vi "Store Configuration Parameters.vi"(8 "error in (no error)":errorcluster, 10 "refnum":T1, 11 "Example Configuration Dialog in":refnum<class "Motor Configuration.lvclass">) -> (0 "error out":errorcluster, 2 "refnum out":T1, 3 "Example Configuration Dialog out":refnum<class "Motor Configuration.lvclass">)   [LabVIEW 2016, in "Hardware.lvlib" / "Motor.lvlib" / "Motor Configuration.lvclass"]
uses:
  <userlib>/Common Components/Hardware/Motor/Motor Config/Motor Configuration.lvclass
  <vilib>/Utility/config.llb/Config Data RefNum.ctl
  <userlib>/Common Components/Hardware/Motor/Motor/Motor.lvclass/Motor.ctl
  <userlib>/Common Components/Hardware/Abstract Hardware/Hardware.lvclass/Hardware.ctl
  <userlib>/Common Components/Hardware/DevInfo/DevInfo.lvclass/DevInfo.ctl
  <userlib>/Common Components/Hardware/Abstract Hardware/Read Label.vi
  <userlib>/Common Components/Hardware/Abstract Hardware/Read DevInfo.vi
  <userlib>/Common Components/Hardware/DevInfo/Read HW Type.vi
  <userlib>/Common Components/Hardware/DevInfo/Read Device Name.vi
  <userlib>/Common Components/Hardware/DevInfo/Read COMM Address.vi
  <userlib>/Common Components/Hardware/DevInfo/Read Sub-COMM Address.vi
  <userlib>/Common Components/Hardware/Motor/Motor/Motor.lvclass
  C:/Program Files (x86)/National Instruments/LabVIEW 2016/user.lib/Common Components/Hardware/Abstract Hardware/Hardware.lvclass
  <userlib>/Common Components/Hardware/Motor/Motor Config/Accessors/Read Motor Obj.vi
  <userlib>/Common Components/Hardware/DevInfo/DevInfo.lvclass
  <vilib>/Utility/config.llb/NI_LVConfig.lvlib
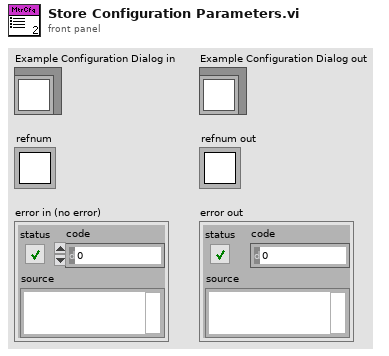
[diagram p1: front panel]
types:
  T1 = typedef "NI_LVConfig.lvlib/Config Data RefNum.ctl" = refnum<k1>
  T2 = typedef "Hardware.lvlib/Motor.lvlib/Motor.lvclass/Motor_Parameters.ctl" = cluster{"closed loop?":bool, "encoder?":bool, "min speed":dbl, "max speed":dbl, "acc time (s)":dbl, "dec time (s)":dbl, "unit mode":enum16{"motor pulses", "real world"}, "motor pulses per revolution":dbl, "display units per motor rev":dbl, "encoder units ratio":dbl, "display unit":string, "display precision":u8, "soft limit min":dbl, "soft limit max":dbl, "Max No. of pull-ins":u8, "Limit+":bool, "Limit+ Logic":enum16{"Low", "High"}, "Limit+ Mode":enum16{"Stop immediately", "Decelerate to Stop"}, "Limit-":bool, "Limit- Logic":enum16{"Low", "High"}, "Limit- Mode":enum16{"Stop immediately", "Decelerate to Stop"}, "Limit+ Sensor ID":enum16{"N/A", "S1", "S2", "S3"}, "Limit- Sensor ID":enum16{"N/A", "S1", "S2", "S3"}, "backlash Compensation":dbl, "soft offset":dbl, "backlash option":enum16{"None", "arriving in + direction", "arriving in - direction"}, "encoder type":enum16{"Linear", "Rotary"}}
  T3 = typedef "Hardware.lvlib/Motor.lvlib/Motor.lvclass/Home Params.ctl" = cluster{"Home Mode":T4, "Home Dir":T5, "Home Pos Shift":dbl}
  T4 = typedef "Hardware.lvlib/Motor.lvlib/Motor.lvclass/Home Mode.ctl" = enum16{"EZ+EL", "EZ only"}
  T5 = typedef "Hardware.lvlib/Motor.lvlib/Motor.lvclass/Home Dir.ctl" = enum16{"negative-", "positive+"}
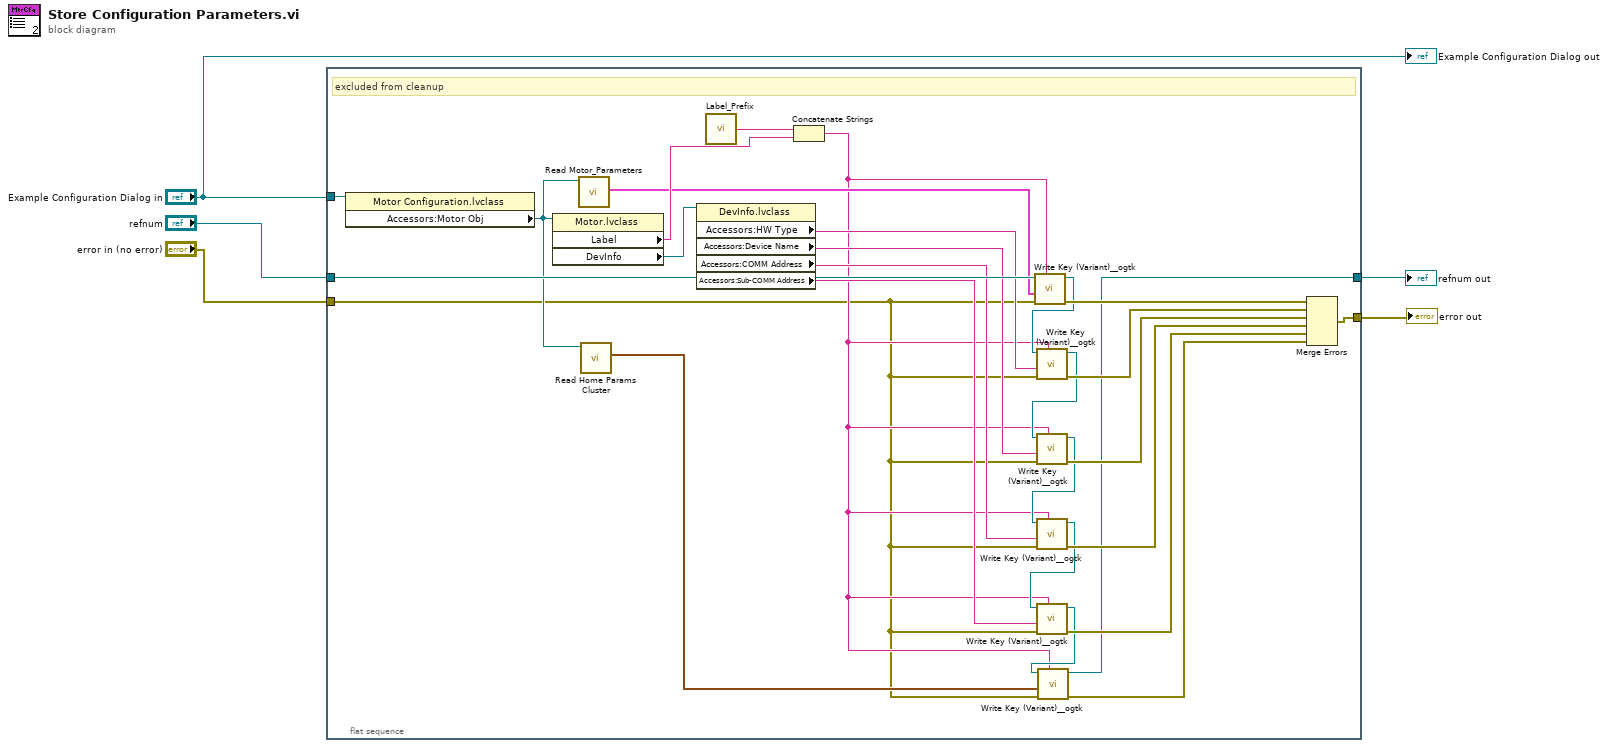
[diagram p0: block diagram]
diagram:
  n1 = flat-sequence {
    tunnel: "refnum" -> [w32]
    tunnel: "error in (no error)" -> [w7]
    tunnel: "Example Configuration Dialog in" -> [w31]
    tunnel: [w10] -> w2
    tunnel: [w30] -> w1
    frame #0 {
      # "excluded from cleanup"
      n2 = property class="Motor Configuration.lvclass"(reference=w31) -> ("Accessors:Motor Obj"=w12:refnum<class "Motor.lvclass">)  [unwired: 1 in, 2 out]
      n3 = property class="Motor.lvclass"(reference=w12) -> ("Label"=w19:string, "DevInfo"=w18:refnum<class "DevInfo.lvclass">)  [unwired: 1 in, 2 out]
      n4 = call <userlib>:"Read Motor_Parameters.vi"("Motor in"=w12) -> ("motor parameters"=w17:T2)  [unwired: 8 in, 2 out]
      n5 = call <userlib>:"Read Home Params Cluster.vi"("Motor in"=w12) -> ("Home Params Cluster"=w8:T3)  [unwired: 8 in, 2 out]
      n6 = property class="DevInfo.lvclass"(reference=w18) -> ("Accessors:HW Type"=w16:string, "Accessors:Device Name"=w15:string, "Accessors:COMM Address"=w14:string, "Accessors:Sub-COMM Address"=w13:string)  [unwired: 1 in, 2 out]
      n7 = call <userlib>:"Label_Prefix.vi"() -> ("Label Prefix String"=w29:string)
      n8 = Concatenate Strings(w29, w19) -> (w9:string)
      n9 = call <userlib>:"Write Key (Variant)__ogtk.vi"("section"=w9, "error in (no error)"=w7, "key-value"=w17, "refnum"=w32) -> ("error out"=w28:errorcluster, "refnum out"=w23:T1)  [unwired: 6 in]
      n10 = call <userlib>:"Write Key (Variant)__ogtk.vi"("section"=w9, "error in (no error)"=w7, "key-value"=w16, "refnum"=w23) -> ("error out"=w27:errorcluster, "refnum out"=w22:T1)  [unwired: 6 in]
      n11 = call <userlib>:"Write Key (Variant)__ogtk.vi"("section"=w9, "error in (no error)"=w7, "key-value"=w15, "refnum"=w22) -> ("error out"=w26:errorcluster, "refnum out"=w21:T1)  [unwired: 6 in]
      n12 = call <userlib>:"Write Key (Variant)__ogtk.vi"("section"=w9, "error in (no error)"=w7, "key-value"=w14, "refnum"=w21) -> ("error out"=w25:errorcluster, "refnum out"=w20:T1)  [unwired: 6 in]
      n13 = call <userlib>:"Write Key (Variant)__ogtk.vi"("section"=w9, "error in (no error)"=w7, "key-value"=w13, "refnum"=w20) -> ("error out"=w24:errorcluster, "refnum out"=w11:T1)  [unwired: 6 in]
      n14 = call <userlib>:"Write Key (Variant)__ogtk.vi"("section"=w9, "error in (no error)"=w7, "key-value"=w8, "refnum"=w11) -> ("error out"=w6:errorcluster, "refnum out"=w10:T1)  [unwired: 6 in]
      n15 = Merge Errors(w28, w27, w26, w25, w24, w6) -> (w30:errorcluster)
    }
  }
  "Example Configuration Dialog out" <- "Example Configuration Dialog in"
  "error out" <- w1
  "refnum out" <- w2
